vi "Add Addr Byte.vi"(8 "error in (no error)":errorcluster, 9 "Slave address":u8 format="%.0x", 10 "Bus operation":T1, 11 "I2C waveform info":T2) -> (0 "error out":errorcluster, 3 "I2C waveform info out":T2)   [LabVIEW 2009, in "IDW.lvlib"]
doc: "Adds a byte containing the <b>Slave address</b> and the \"Read/not Write\" bit to the I2C waveform. The \"Read/not Write\" bit is '0' for a <b>Transmit (Tx)</b> Bus operation and '1' for a <b> Receive (Rx)</b> operation.\n\nEach bit of the Slave address is added in the <b>Byte order</b> order. Only the first 7 bits of the Slave address value are used. The 8th bit is replaced by the \"Read/not Write\" bit. For each bit, the value is written to the SDA line according to the timing parameters specified by the <b>Init</b> VI.\n\nTiming parameters that affect this waveform segment's length are: <b>tSU;DAT</b>, <b>tHIGH</b>, and <b>tHD;DAT</b>."
uses:
  IDW.lvlib
  _Typedefs/Waveform info.ctl
  _Typedefs/Timing - ticks.ctl
  _Typedefs/Default transition action.ctl
  _Typedefs/Bit type.ctl
  _Typedefs/Bus operation.ctl
  _Polymorphics/Interpret Data - Byte.vi
  _Typedefs/Byte order.ctl
  _Typedefs/Transition action.ctl
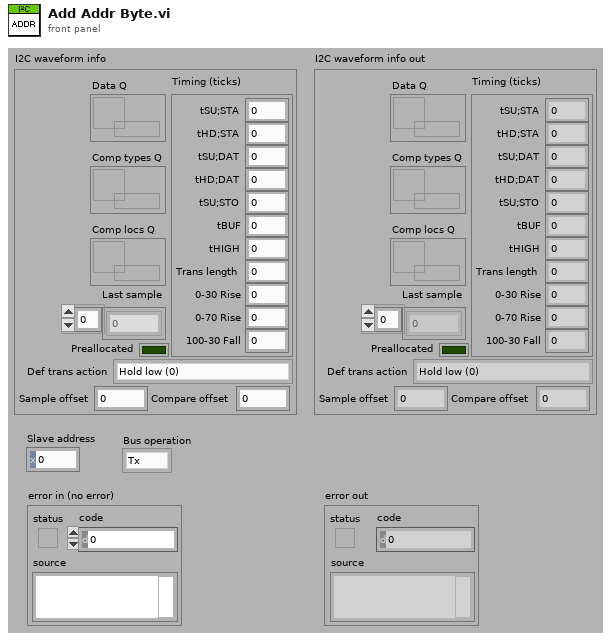
[diagram p1: front panel]
types:
  T1 = typedef "IDW.lvlib/Bus operation.ctl" = enum16{"Tx", "Rx"}
  T2 = typedef "IDW.lvlib/Waveform info.ctl" = cluster{"Last sample":u8[], "Sample offset":u64, "Compare offset":u64, "Timing (ticks)":T3, "Preallocated":bool, "Def trans action":T4, "Data Q":refnum<queue>, "Comp types Q":refnum<queue>, "Comp locs Q":refnum<queue>}
  T3 = typedef "IDW.lvlib/Timing - ticks.ctl" = cluster{"tSU;STA":i32, "tHD;STA":i32, "tSU;DAT":i32, "tHD;DAT":i32, "tSU;STO":i32, "tBUF":i32, "tHIGH":i32, "Trans length":i32, "0-30 Rise":i32, "0-70 Rise":i32, "100-30 Fall":i32}
  T4 = typedef "IDW.lvlib/Default transition action.ctl" = enum16{"Hold low (0)", "Release (Z)", "Set up next value", "Hold previous value", "Preserve tHD;DAT and tSU;DAT"}
  T5 = typedef "IDW.lvlib/Byte order.ctl" = enum16{"MSB", "LSB"}
  T6 = typedef "IDW.lvlib/Transition action.ctl" = enum16{"Hold low (0)", "Release (Z)", "Set up next value", "Hold previous value", "Preserve tHD;DAT and tSU;DAT", "<Use session default>"}
  T7 = typedef "IDW.lvlib/Bit type.ctl" = enum16{"ACK", "Data"}
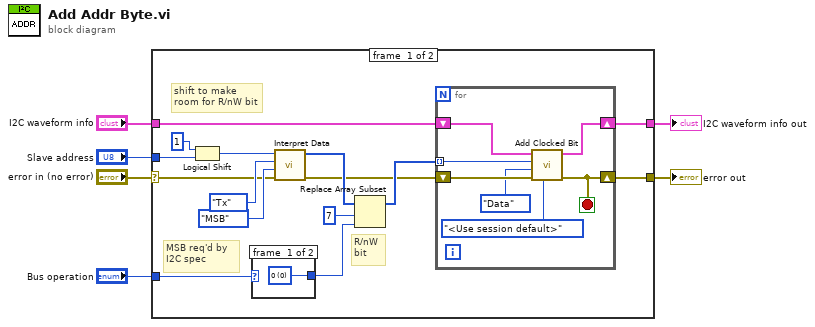
[diagram p0: block diagram]
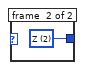
[diagram p2: hidden frame]
diagram:
  n1 = case shown="No Error" "error in (no error)" {
    selector: "error in (no error)" -> [w8 w32]
    tunnel: "Slave address" -> [w11 _]
    tunnel: [w15 w31] -> w5
    tunnel: "I2C waveform info" -> [w16 w31]
    tunnel: "Bus operation" -> [w18 _]
    tunnel: [w17 w32] -> w1
    frame #0 {
      # "MSB req'd by I2C spec"
      # "shift to make room for R/nW bit"
      # "R/nW\nbit"
      n2 = Logical Shift(y=i8 1, x=w11) -> (x << y=w9:u8)
      n3 = case shown="\"Rx\"" w18 {
        tunnel: [w22 w23] -> w20
        frame #0 {
          w22 = u8 0 items=["0", "1", "Z", "L", "H", "X", "T", "V"] ("Bit")
        }
        frame #1 {
          w23 = u8 2 items=["0", "1", "Z", "L", "H", "X", "T", "V"] ("Bit")
        }
      }
      n4 = call-poly "Interpret Data.vi"("error in (no error)"=w8, "Byte order"=Byte_order."MSB", "Action"=Bus_operation."Tx", "Data"=w9) -> ("error out"=w7:errorcluster, "Digital data bits"=w14:u8[])  [unwired: 6 out]
      n5 = Replace Array Subset(array=w14, new element=w20, index=7) -> (w21:u8[])
      n6 = for {
        shift-right: [w29] -> w15
        shift-left: w16 -> [w30]
        tunnel: w21 -> [w28] mode=indexing
        shift-right: [w26] -> w17
        shift-left: w7 -> [w27]
        stop <- w26 stop-if-true
        n7 = call "Add Clocked Bit.vi"("Transition action"=Transition_action."<Use session default>", "error in (no error)"=w27, "Bit type"=Bit_type."Data", "Bit value"=w28, "I2C waveform info"=w30) -> ("error out"=w26:errorcluster, "I2C waveform info out"=w29:T2)  [unwired: 5 out]
      }
    }
    frame #1 {
    }
  }
  "I2C waveform info out" <- w5
  "error out" <- w1
